vi "subOpenAppBuilderVI.vi"(8 "error in (no error)":errorcluster, 11 "Application in":refnum<vi>) -> (0 "error out":errorcluster, 3 "VI ref":refnum<vi>)   [LabVIEW 2020, in "SolutionBuilder.lvlib" / "BuildManager.lvclass"]
uses:
  BuildManager.lvclass
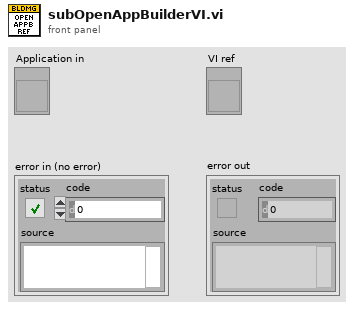
[diagram p1: front panel]
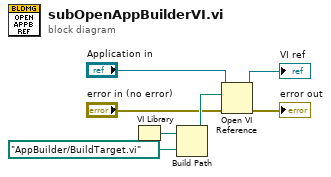
[diagram p0: block diagram]
diagram:
  n1 = VI Library() -> (path=w4:path)
  n2 = Build Path(base path=w4, name or relative path=path "AppBuilder/BuildTarget.vi" ("vi path")) -> (appended path=w6:path)
  n3 = Open VI Reference(application reference (local)="Application in", vi path=w6, error in (no error)="error in (no error)") -> (vi reference=→"VI ref":refnum<vi>, error out=→"error out":errorcluster)  [unwired: 1 in, 2 out]
